vi "Error Handling.vi"() -> ()   [LabVIEW 2020]
uses:
  <vilib>/DAQmx/read.llb/DAQmx Read (Analog 2D DBL NChan NSamp).vi
  <vilib>/DAQmx/create/channels.llb/DAQmx Create Channel (AI-Acceleration-Accelerometer).vi
  <vilib>/DAQmx/configure/timing.llb/DAQmx Timing (Sample Clock).vi
  <vilib>/DAQmx/miscellaneous.llb/DAQmx Fill In Error Info.vi
panel:
  out "Acceleration Data - Graph":dbl[][](graph)
  out "Acceleration Data - Array":dbl[][](array[numeric])
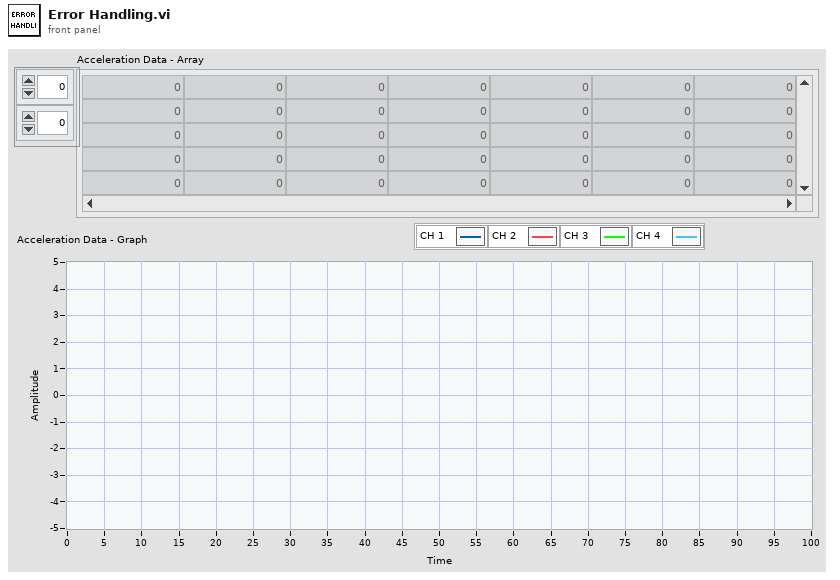
[diagram p1: front panel]
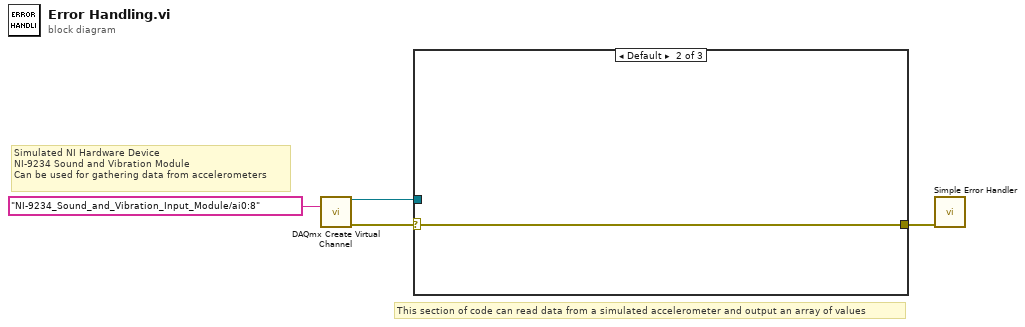
[diagram p0: block diagram]
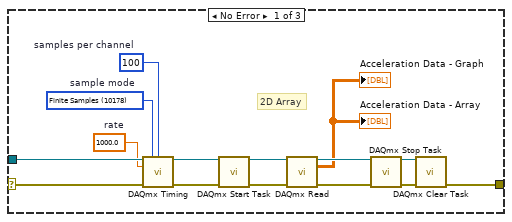
[diagram p2: hidden frame]
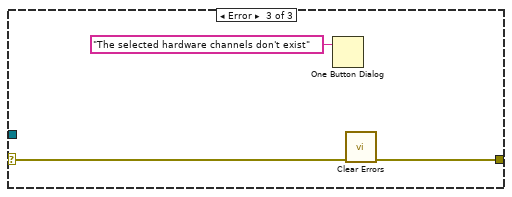
[diagram p3: hidden frame]
diagram:
  # "This section of code can read data from a simulated accelerometer and output an array of values"
  # "Simulated NI Hardware Device\nNI-9234 Sound and Vibration Module\nCan be used for gathering data from accelerometers"
  n1 = call-poly <vilib>:"DAQmx Create Virtual Channel.vi"("physical channels"=tag "NI-9234_Sound_and_Vibration_Input_Module/ai0:8") -> ("task out"=w3:refnum<k21>, "error out"=w2:errorcluster)  [unwired: 13 in]
  n2 = case shown="Default" w2 {
    selector: w2 -> [w12 w20 w22]
    tunnel: w3 -> [w13 _ _]
    tunnel: [w5 w20 w21] -> w1
    frame No Error {
      w7 = 1000.0  # rate
      w8 = 100  # samples per channel
      w9 = 10178 items=["Finite Samples"=10178, "Continuous Samples"=10123, "Hardware Timed Single Point"=12522]  # sample mode
      # "2D Array"
      n3 = call-poly <vilib>:"DAQmx Timing.vi"("task/channels in"=w13, "sample mode"=w9, "samples per channel"=w8, "rate"=w7, "error in"=w12) -> ("task out"=w11:refnum<k21>, "error out"=w10:errorcluster)  [unwired: 9 in]
      n4 = call <vilib>:"DAQmx Start Task.vi"("task/channels in"=w11, "error in"=w10) -> ("task out"=w18:refnum<k21>, "error out"=w19:errorcluster)  [unwired: 12 in]
      n5 = call-poly <vilib>:"DAQmx Read.vi"("task/channels in"=w18, "error in"=w19) -> ("task out"=w16:refnum<k21>, "data"=→"Acceleration Data - Array" →"Acceleration Data - Graph":dbl[][], "error out"=w15:errorcluster)  [unwired: 11 in]
      n6 = call <vilib>:"DAQmx Stop Task.vi"("task/channels in"=w16, "error in"=w15) -> ("task out"=w17:refnum<k21>, "error out"=w14:errorcluster)  [unwired: 12 in]
      n7 = call <vilib>:"DAQmx Clear Task.vi"("task in"=w17, "error in"=w14) -> ("error out"=w5:errorcluster)  [unwired: 13 in]
    }
    frame Default {
    }
    frame Error {
      n8 = One Button Dialog(message="The selected hardware channels don't exist") -> ()  [unwired: 1 in, 1 out]
      n9 = call <vilib>:"Clear Errors.vi"("error in (no error)"=w22) -> ("error out"=w21:errorcluster)  [unwired: 5 in, 1 out]
    }
  }
  n10 = call <vilib>:"Simple Error Handler.vi"("error in (no error)"=w1) -> ()  [unwired: 4 in, 5 out]
